vi "Initialize Function Actor Core.vi"(5 "Cmd List":refnum<vi>, 7 "Connected Clients":refnum<vi>, 8 "error in (no error)":errorcluster, 11 "Function in":refnum<class "Function.lvclass">) -> (0 "error out":errorcluster, 1 "event out":refnum<user-event>, 2 "notifier out":refnum<notifier>, 3 "Function out":refnum<class "Function.lvclass">)   [LabVIEW 2016, in "Function Actor.lvlib" / "Function.lvclass"]
uses:
  <userlib>/Common Components/Function Actor/Function.lvclass
  C:/Program Files (x86)/National Instruments/LabVIEW 2016/vi.lib/ActorFramework/Actor/Actor.lvclass
  <userlib>/Common Components/Function Actor/Function.lvclass/Function.ctl
  <vilib>/ActorFramework/Actor/Actor.lvclass/Actor.ctl
  <vilib>/ActorFramework/Message Enqueuer/Message Enqueuer.lvclass/Message Enqueuer.ctl
  <userlib>/Common Components/Function Actor/Accessors/Read Not legacy_.vi
  <vilib>/ActorFramework/Message Enqueuer/Init from Existing Queue.vi
  <vilib>/ActorFramework/Message Enqueuer/Enqueue.vi
  <userlib>/Common Components/Function Messages/Initialize Msg/Initialize Msg.lvclass
  C:/Program Files (x86)/National Instruments/LabVIEW 2016/vi.lib/ActorFramework/Message/Message.lvclass
  <userlib>/Common Components/Function Actor/Messages/Configure Msg/Configure Msg.lvclass
  <vilib>/ActorFramework/Message Priority Queue/Priority Enqueue.vi
  <vilib>/ActorFramework/Message Enqueuer/Message Enqueuer.lvclass
  <vilib>/ActorFramework/Actor/Actor.lvclass
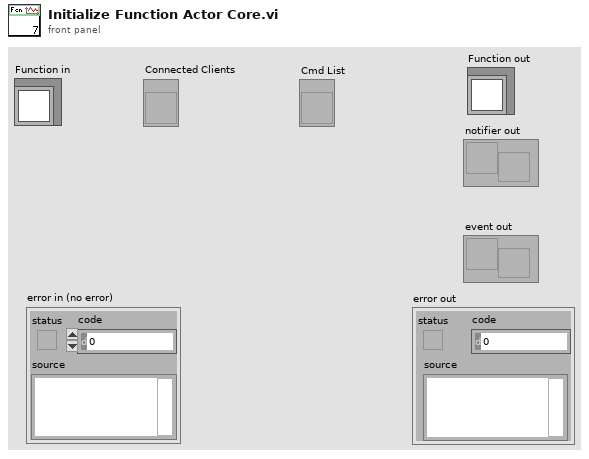
[diagram p1: front panel]
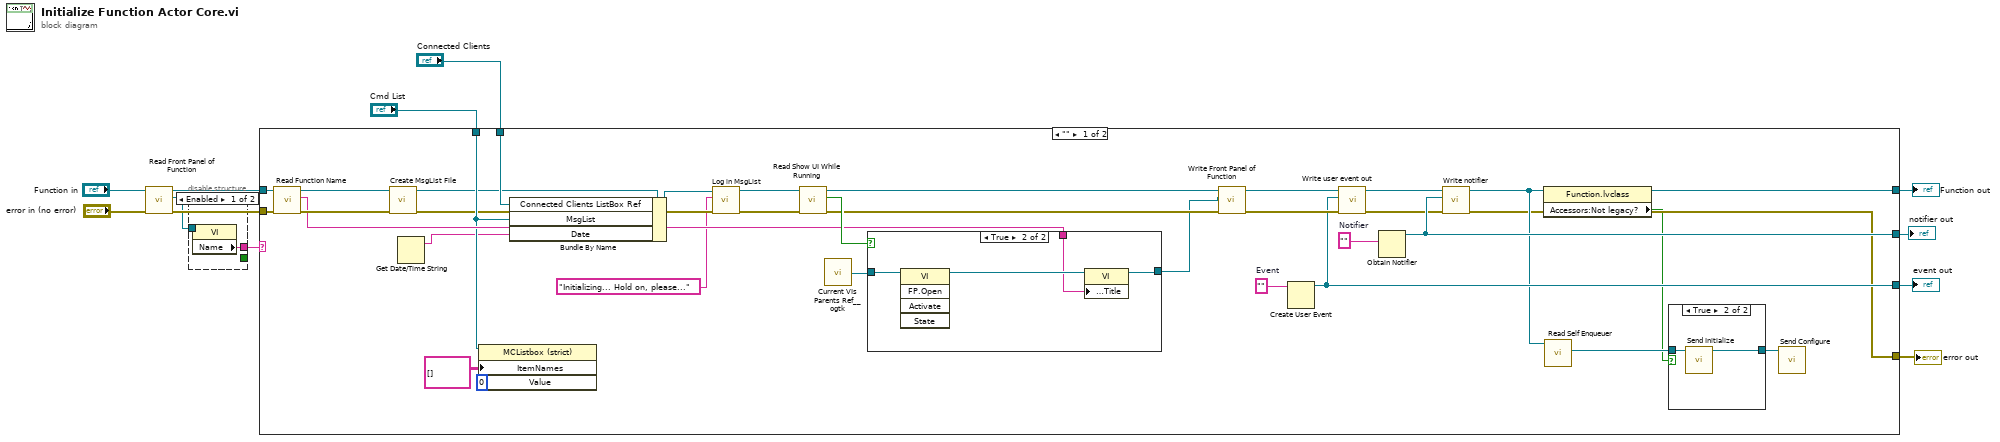
[diagram p0: block diagram]
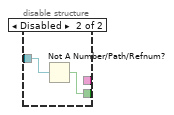
[diagram p2: hidden frame]
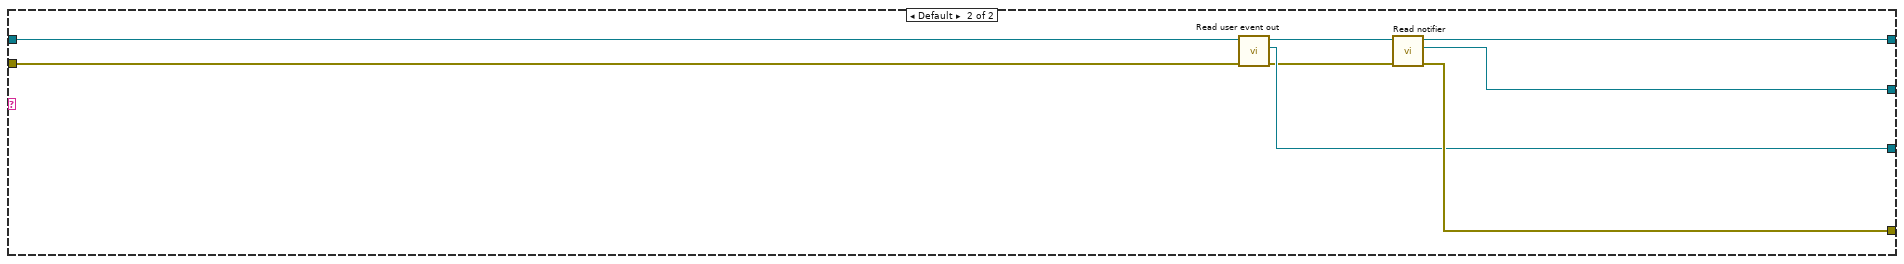
[diagram p5: hidden frame]
diagram:
  n1 = call <userlib>:"Read Front Panel of Function.vi"("error in (no error)"="error in (no error)", "Function in"="Function in") -> ("error out"=w11:errorcluster, "Front Panel of Function"=w3:refnum<vi>, "Function out"=w12:refnum<class "Function.lvclass">)  [unwired: 7 in]
  n2 = disable-structure shown="Enabled" {
    disable-tunnel: w3 -> [w14 w16]
    disable-tunnel: [w13 _] -> w4
    disable-tunnel: [_ w15] -> _
    frame Enabled {
      n3 = property class="VI"(reference=w14) -> ("Name"=w13:string)  [unwired: 1 in, 2 out]
    }
    frame Disabled {
      n4 = Not A Number/Path/Refnum?(number/path/refnum=w16) -> (NaN/Path/Refnum?=w15:bool)
    }
  }
  n5 = case shown="\"\"" w4 {
    tunnel: [w32 w67] -> w9
    tunnel: w12 -> [w28 w64]
    tunnel: w11 -> [w40 w61]
    tunnel: [w50 w66] -> w10
    tunnel: [w36 w65] -> w8
    tunnel: [w41 w62] -> w7
    tunnel: "Cmd List" -> [w26 _]
    tunnel: "Connected Clients" -> [w25 _]
    frame "" {
      w46 = ""  # Event
      w51 = ""  # Notifier
      n6 = call <userlib>:"Read Function Name.vi"("error in (no error)"=w40, "Function in"=w28) -> ("error out"=w29:errorcluster, "Function Name"=w27:string, "Function out"=w23:refnum<class "Function.lvclass">)  [unwired: 7 in]
      n7 = call <userlib>:"Create MsgList File.vi"("error in (no error)"=w29, "Function in"=w23) -> ("error out"=w24:errorcluster, "Function out"=w22:refnum<class "Function.lvclass">)  [unwired: 8 in]
      n8 = Get Date/Time String() -> (date string=w21:string)  [unwired: 3 in, 1 out]
      n9 = property class="MCListbox (strict)"(reference=w26, "ItemNames"=string[][] [] ("Item Names"), "Value"=0) -> ()  [unwired: 1 in, 2 out]
      n10 = Bundle By Name(cluster=w22, "Connected Clients ListBox Ref"=w25, "MsgList"=w26, "Date"=w21) -> (w19:refnum<class "Function.lvclass">)
      n11 = call-dynamic "Log in MsgList.vi"("error in (no error)"=w24, "Msg"="Initializing... Hold on, please...", "Function in"=w19) -> ("error out"=w20:errorcluster, "Function out"=w18:refnum<class "Function.lvclass">)  [unwired: 7 in]
      n12 = call <userlib>:"Read Show UI While Running.vi"("error in (no error)"=w20, "Function in"=w18) -> ("error out"=w47:errorcluster, "Show UI While Running"=w49:bool, "Function out"=w48:refnum<class "Function.lvclass">)  [unwired: 7 in]
      n13 = call <userlib>:"Current VIs Parents Ref__ogtk.vi"() -> ("Calling VI's Reference"=w33:refnum<vi>)  [unwired: 2 in]
      n14 = case shown="True" w49 {
        tunnel: w33 -> [w55 w59]
        tunnel: [w55 w57] -> w34
        tunnel: w27 -> [_ w56]
        frame False {
        }
        frame True {
          n15 = invoke class="VI" method="FP.Open"(reference=w59) -> (reference out=w58:refnum<vi>)  [unwired: 4 in, 4 out]
          n16 = property class="VI"(reference=w58, "Front Panel.Title"=w56) -> (reference out=w57:refnum<vi>)  [unwired: 1 in, 1 out]
        }
      }
      n17 = call <userlib>:"Write Front Panel of Function.vi"("error in (no error)"=w47, "Front Panel of Function"=w34, "Function in"=w48) -> ("error out"=w43:errorcluster, "Function out"=w45:refnum<class "Function.lvclass">)  [unwired: 7 in]
      n18 = Create User Event(user event datatype=w46) -> (user event=w41:refnum<user-event>)  [unwired: 1 in, 1 out]
      n19 = call <userlib>:"Write user event out.vi"("error in (no error)"=w43, "user event out"=w41, "Function in"=w45) -> ("error out"=w42:errorcluster, "Function out"=w44:refnum<class "Function.lvclass">)  [unwired: 7 in]
      n20 = Obtain Notifier(notification data type=w51) -> (notifier out=w50:refnum<notifier>)  [unwired: 3 in, 2 out]
      n21 = call <userlib>:"Write notifier.vi"("error in (no error)"=w42, "notifier"=w50, "Function in"=w44) -> ("error out"=w36:errorcluster, "Function out"=w37:refnum<class "Function.lvclass">)  [unwired: 7 in]
      n22 = property class="Function.lvclass"(reference=w37) -> (reference out=w32:refnum<class "Function.lvclass">, "Accessors:Not legacy?"=w30:bool)  [unwired: 1 in, 1 out]
      n23 = call <vilib>:"Read Self Enqueuer.vi"("Actor"=w37) -> ("Self Enqueuer"=w35:refnum<class "Message Enqueuer.lvclass">)  [unwired: 10 in]
      n24 = case shown="True" w30 {
        tunnel: w35 -> [w52 w54]
        tunnel: [w52 w53] -> w31
        frame False {
        }
        frame True {
          n25 = call <userlib>:"Send Initialize.vi"("Message Enqueuer"=w54) -> ("Message Enqueuer out"=w53:refnum<class "Message Enqueuer.lvclass">)  [unwired: 9 in, 1 out]
        }
      }
      n26 = call <userlib>:"Send Configure.vi"("Message Enqueuer in"=w31) -> ()  [unwired: 9 in, 2 out]
    }
    frame Default {
      n27 = call <userlib>:"Read user event out.vi"("error in (no error)"=w61, "Function in"=w64) -> ("error out"=w60:errorcluster, "user event out"=w62:refnum<user-event>, "Function out"=w63:refnum<class "Function.lvclass">)  [unwired: 7 in]
      n28 = call <userlib>:"Read notifier.vi"("error in (no error)"=w60, "Function in"=w63) -> ("error out"=w65:errorcluster, "notifier"=w66:refnum<notifier>, "Function out"=w67:refnum<class "Function.lvclass">)  [unwired: 7 in]
    }
  }
  "Function out" <- w9
  "error out" <- w8
  "notifier out" <- w10
  "event out" <- w7
